vi "SVT Shock Response Spectrum (1 Ch - N Max Types).vi"(0 "scaled signal [EU]":waveform(dbl), 1 "maximum value types":i32[](array[ring])=[0] items=["Maximax", "Initial positive", "Initial negative", "Initial absolute", "Residual positive", "Residual negative", "Residual absolute"], 2 "pulse duration [ms]":dbl=-1.0 format="%.2f", 5 "frequency range":T1={"low frequency [Hz]"=10.0, "high frequency [Hz]"=100.0, "frequencies / octave"=6} {"high frequency [Hz]" format="%.2f"; "low frequency [Hz]" format="%.2f"}, 7 "model":i32(ring) items=["Absolute acceleration", "Relative displacement"], 9 "critical damping factor":dbl=0.05 format="%.2f", 11 "error in (no error)":errorcluster, 12 "preprocessing settings":T2 {"lowpass cutoff frequency [Hz]" format="%.2f"}, 13 "desired units":i32(ring)=-1 items=["no change"=-1, "m/s^2"=0, "mm/s^2"=2, "micron/s^2"=3, "in/s^2"=1, "mil/s^2"=5]) -> (4 "shock spectra":T3(array[cluster]) {"maximum values" format="%.2f"; "natural frequencies [Hz]" format="%.2f"}, 6 "unit label":string, 15 "error out":errorcluster)   [LabVIEW 2017, in "SoundVib_Transient.lvlib"]
doc: "Computes the peak levels for each single-degree-of-freedom (SDOF) component to form the shock response spectrum (SRS) across the <B>frequency range</B> of interest. Wire data to the <B>scaled signal [EU]</B> input to determine the polymorphic instance to use or manually select the instance."
uses:
  <vilib>/addons/Sound and Vibration/svt_Transients/SoundVib_Transient.lvlib
  <vilib>/addons/_NISVFA/_Shared subVIs/Common/svc_Engineering Units to Unit Label.vi
  <vilib>/addons/_NISVFA/_Shared subVIs/Common/svc_Unit Label to Engineering Units.vi
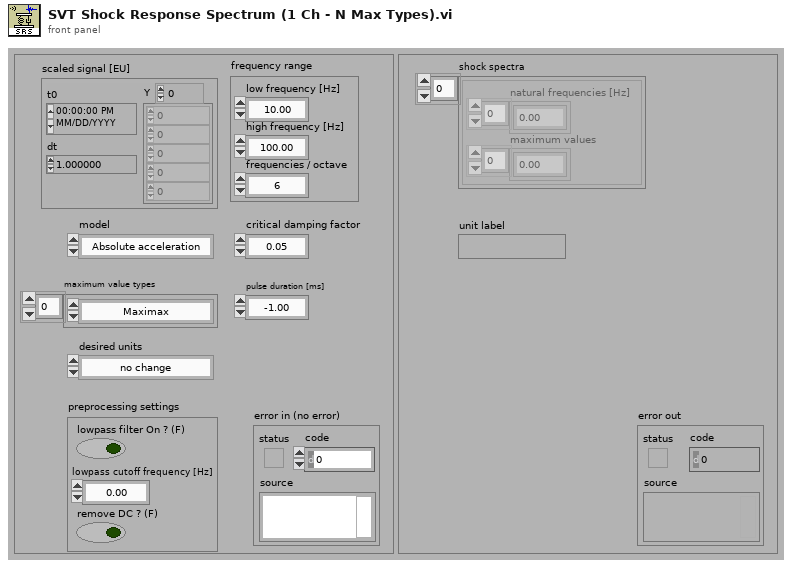
[diagram p1: front panel]
types:
  T1 = cluster{"low frequency [Hz]":dbl, "high frequency [Hz]":dbl, "frequencies / octave":i32}
  T2 = cluster{"lowpass filter On ? (F)":bool, "lowpass cutoff frequency [Hz]":dbl, "remove DC ? (F)":bool}
  T3 = cluster{"natural frequencies [Hz]":dbl[], "maximum values":dbl[]}[]
  T4 = cluster{"natural frequencies [Hz]":dbl[], dbl[]}[]
  T5 = typedef "svc_Channel Info.ctl" = cluster{"sensor sensitivity":dbl, "engineering units":T6, "dB reference":dbl, "custom label":string, "weighting filter":T7, "pregain":dbl}
  T6 = typedef "svc_Engineering Units Text Ring.ctl" = u16
  T7 = typedef "svc_Weighting Filter Text Ring.ctl" = u16
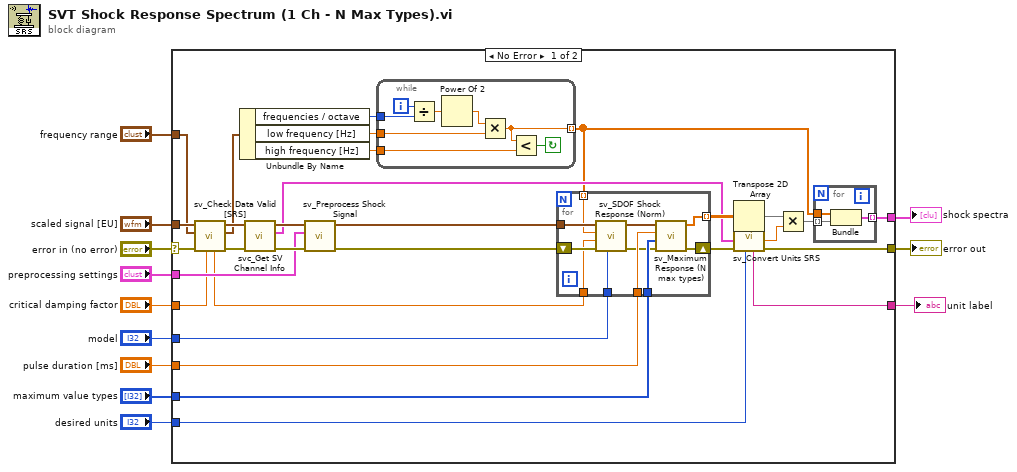
[diagram p0: block diagram]
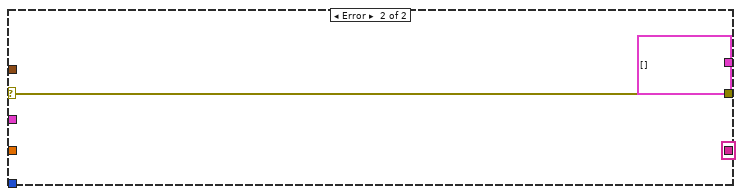
[diagram p2: hidden frame]
diagram:
  n1 = case shown="No Error" "error in (no error)" {
    selector: "error in (no error)" -> [w26 w67]
    tunnel: [w35 w67] -> w11
    tunnel: "scaled signal [EU]" -> [w27 _]
    tunnel: "preprocessing settings" -> [w31 _]
    tunnel: "frequency range" -> [w25 _]
    tunnel: "pulse duration [ms]" -> [w39 _]
    tunnel: [w38 T4 []] -> w6
    tunnel: "critical damping factor" -> [w24 _]
    tunnel: "model" -> [w34 _]
    tunnel: "maximum value types" -> [w37 _]
    tunnel: [w21 "" ("unit label")] -> w2
    tunnel: "desired units" -> [w22 _]
    frame No Error {
      n2 = call <vilib>:"sv_Check Data Valid [SRS].vi"("critical damping factor"=w24, "error in (no error)"=w26, "frequency range"=w25, "scaled signal [EU]"=w27) -> ("error out"=w29:errorcluster, "dup frequency range"=w14:T1, "dup scaled signal [EU]"=w28:waveform(dbl), "dup critical damping"=w23:dbl)  [unwired: 4 in]
      n3 = Unbundle By Name(w14) -> ("frequencies / octave"=w17:i32, "low frequency [Hz]"=w16:dbl, "high frequency [Hz]"=w15:dbl)
      n4 = call <vilib>:"svc_Get SV Channel Info.vi"("error in (no error)"=w29, "scaled signal [EU]"=w28) -> ("error out"=w32:errorcluster, "channel info"=w30:T5, "dup scaled signal [EU]"=w33:waveform(dbl))  [unwired: 4 in, 3 out]
      n5 = call <vilib>:"sv_Preprocess Shock Signal.vi"("error in (no error)"=w32, "preprocessing settings"=w31, "scaled signal [EU]"=w33) -> ("error out"=w40:errorcluster, "filtered scaled signal [EU]"=w41:waveform(dbl))  [unwired: 7 in]
      n6 = while {
        tunnel: [w43] -> w13 mode=indexing
        tunnel: w15 -> [w45]
        tunnel: w16 -> [w46]
        tunnel: w17 -> [w49]
        i -> [w50]
        stop <- w44 continue-if-true
        n7 = Divide(x=w50, y=w49) -> (x/y=w48:dbl)
        n8 = Power Of 2(x=w48) -> (2^x=w47:dbl)
        n9 = Multiply(x=w47, y=w46) -> (x*y=w43:dbl)
        n10 = Less?(x=w43, y=w45) -> (x < y?=w44:bool)
      }
      n11 = for {
        tunnel: w41 -> [w60]
        tunnel: w23 -> [w58]
        tunnel: w37 -> [w64]
        tunnel: [w62] -> w42 mode=indexing
        tunnel: w34 -> [w57]
        shift-right: [w63] -> w36
        shift-left: w40 -> [w59]
        tunnel: w39 -> [w61]
        tunnel: w13 -> [w54] mode=indexing
        n12 = call <vilib>:"sv_SDOF Shock Response (Norm).vi"("model"=w57, "error in (no error)"=w59, "critical damping factor"=w58, "fn [Hz]"=w54, "scaled signal [EU]"=w60) -> ("error out"=w55:errorcluster, "SDOF shock response"=w56:waveform(dbl))  [unwired: 5 in]
        n13 = call <vilib>:"sv_Maximum Response (N max types).vi"("error in (no error)"=w55, "maximum value types"=w64, "pulse duration [ms]"=w61, "SDOF shock response"=w56) -> ("error out"=w63:errorcluster, "maximum values"=w62:dbl[])  [unwired: 4 in, 2 out]
      }
      n14 = Transpose 2D Array(2D array=w42) -> (transposed array=w20:dbl[][])
      n15 = call <vilib>:"sv_Convert Units SRS.vi"("desired units"=w22, "error in (no error)"=w36, "channel info"=w30) -> ("error out"=w35:errorcluster, "scale factor"=w19:dbl, "unit label"=w21:string)  [unwired: 4 in]
      n16 = Multiply(x=w20, y=w19) -> (x*y=w18:dbl[][])
      n17 = for {
        tunnel: w18 -> [w53] mode=indexing
        tunnel: w13 -> [w52]
        tunnel: [w51] -> w38 mode=indexing
        n18 = Bundle(w52, w53) -> (w51:cluster{dbl[], dbl[]})  [unwired: 1 in]
      }
    }
    frame Error {
    }
  }
  "error out" <- w11
  "shock spectra" <- w6
  "unit label" <- w2
